vi "processing.vi"(0 "Refnum in":T2, 5 "manual crop":bool, 7 "Erode process":bool, 9 "invert":bool) -> (3 "height less than 1cm(80pixels)":bool, 4 "after complete processing":T2, 10 "array of mean":sgl[](array[numeric]), 14 "image features":T3, 15 "Array of SD":sgl[](array[numeric]))   [LabVIEW 2011]
uses:
  <vilib>/vision/Image Controls.llb/IMAQ Image.ctl
  <vilib>/vision/NI_Vision_Development_Module.lvlib
  <vilib>/Analysis/NI_AALBase.lvlib
panel:
  in  "Tab Control":T1(tab)
  out "after invert(optional), crop (optional)":T2(plugin-control)
  out "after theshold":T2(plugin-control)
  out "after scan and make text white":T2(plugin-control)
  out "after particle filter":T2(plugin-control)
  out "after b/w to gray":T2(plugin-control)
  in  "Look For (Threshold 1)":u32(ring) items=["Bright Objects", "Dark Objects"]
  in  "Keep/Remove Particles (Particle Filter 1)":bool=TRUE
  in  "Connectivity 4/8 (8) (Particle Filter 1)":bool=TRUE
  out "subarray":sgl[](array[numeric])
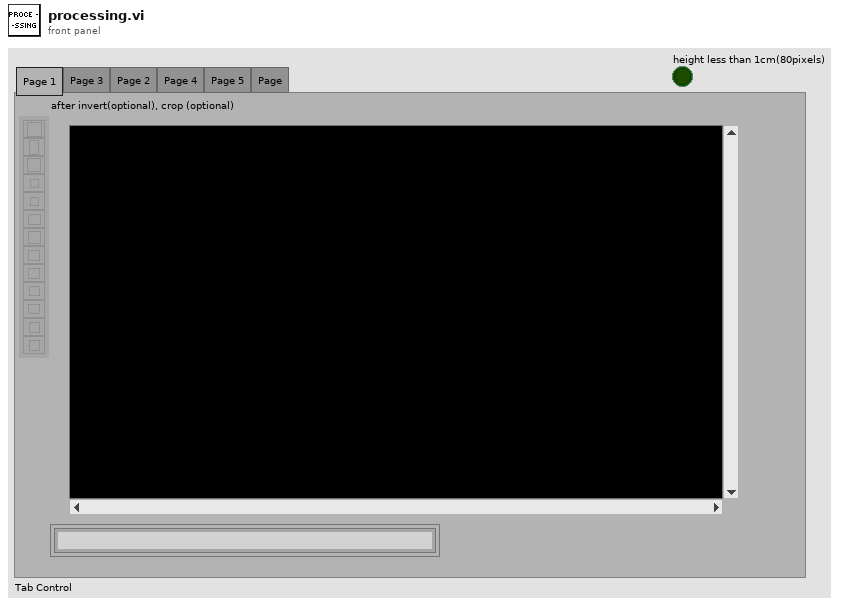
[diagram p1: front panel]
types:
  T1 = enum32{"Page 1", "Page 3", "Page 2", "Page 4", "Page 5", "Page"}
  T2 = typedef "IMAQ Image.ctl" = refnum<image>
  T3 = cluster{"text was :":bool, "top":i32, "bottom":i32}
  T4 = cluster{"Measurement Parameter":i32, "Range Lower Value":dbl, "Range Upper Value":dbl, "Range":bool, "Measurement Type":bool}[]
  T5 = enum32{"AutoM", "Close", "Dilate", "Erode", "Gradient", "Gradient in", "Gradient out", "HitMiss", "Open", "PClose", "POpen", "Thick", "Thin"}
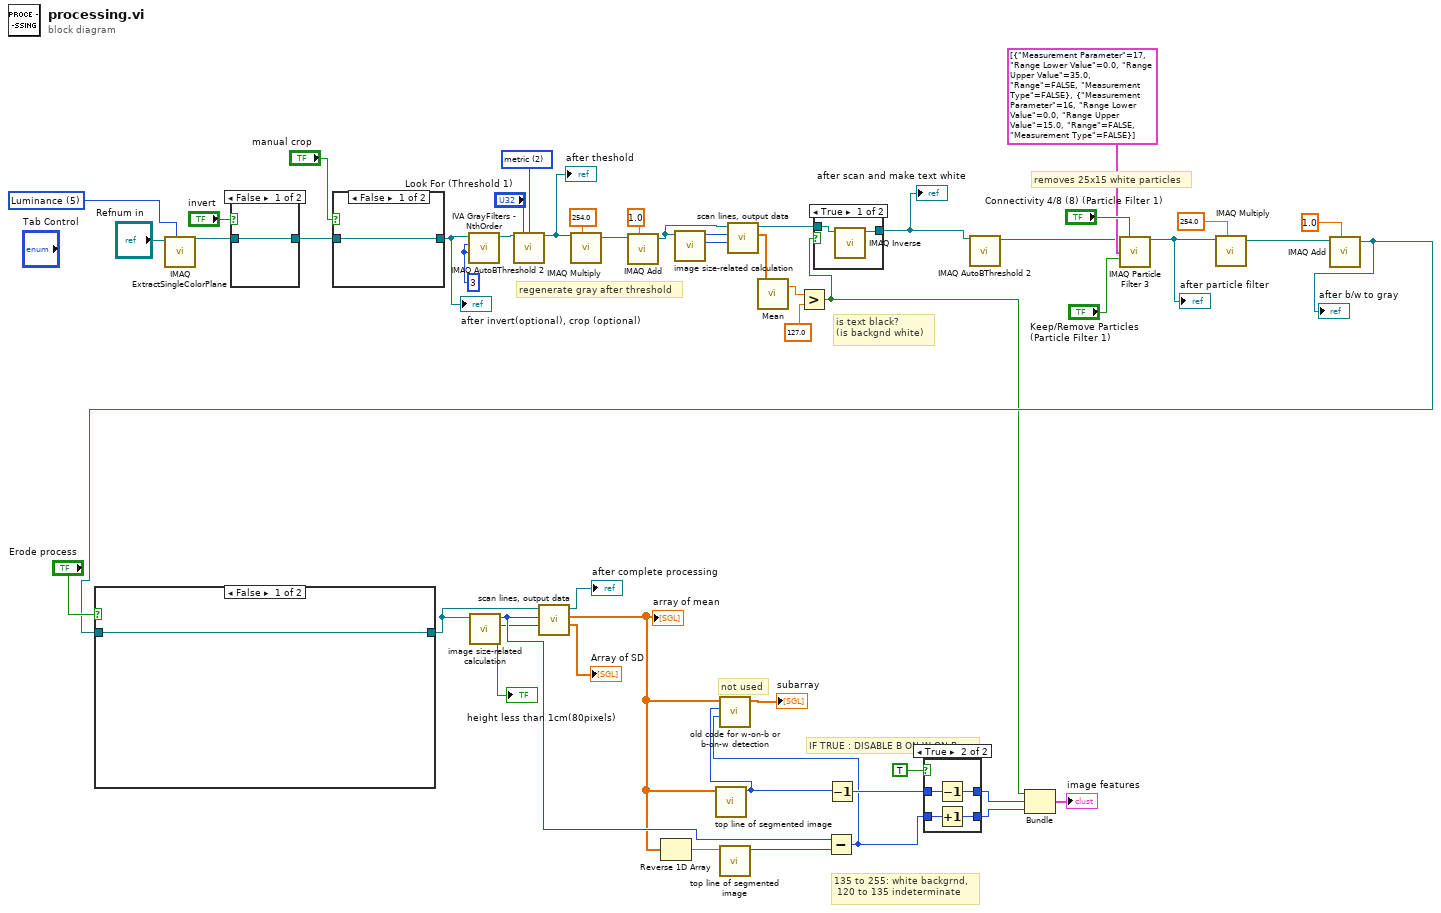
[diagram p0: block diagram]
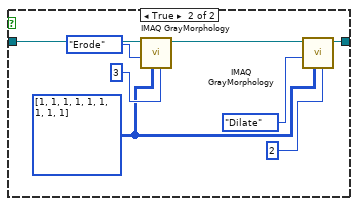
[diagram p4: hidden frame]
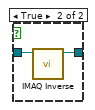
[diagram p5: hidden frame]
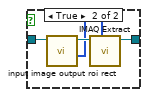
[diagram p6: hidden frame]
diagram:
  w37 = 3 ("Filter size X")
  w44 = 2 items=["clustering", "entropy", "metric", "moments", "inter-class variance"] ("Method (Threshold 1)")
  w47 = 5 items=["Red", "Green", "Blue", "Hue", "Saturation", "Luminance", "Value", "Intensity"] ("Color Plane (Color Plane Extraction 1)")
  # "not used"
  # "is text black?\n(is backgnd white)"
  # "regenerate gray after threshold"
  # "removes 25x15 white particles"
  # "IF TRUE : DISABLE B ON W ON B"
  # "135 to 255: white backgrnd,\n 120 to 135 indeterminate"
  n1 = call "IMAQ ExtractSingleColorPlane"("Color Plane"=w47, "Image Src"="Refnum in") -> ("Image Dst Out"=w49:T2)  [unwired: 2 in, 7 out]
  n2 = case shown="False" "invert" {
    tunnel: w49 -> [w52 w54]
    tunnel: [w52 w53] -> w46
    frame False {
    }
    frame True {
      n3 = call "IMAQ Inverse"("Image Src"=w54) -> ("Image Dst Out"=w53:T2)  [unwired: 9 in, 1 out]
    }
  }
  n4 = case shown="False" "manual crop" {
    tunnel: [w55 w58] -> w10
    tunnel: w46 -> [w55 w57]
    frame False {
    }
    frame True {
      n5 = call "input image output roi rect.vi"("Refnum in"=w57) -> ("selected rectangle"=w56:i32[], "Refnum out"=w59:T2)  [unwired: 9 in]
      n6 = call "IMAQ Extract"("Optional Rectangle"=w56, "Image Src"=w59) -> ("Image Dst Out"=w58:T2)  [unwired: 8 in, 1 out]
    }
  }
  "after invert(optional), crop (optional)" <- w10
  n7 = call <vilib>:"IVA GrayFilters - NthOrder.vi"("Filter size Y"=w37, "Filter size X"=w37, "Image In"=w10) -> ("Image Out"=w36:T2)  [unwired: 1 in, 7 out]
  n8 = call "IMAQ AutoBThreshold 2"("Image Src"=w36, "Look For (Bright Objects)"="Look For (Threshold 1)", "Method (clustering)"=w44) -> ("Image Dst Out"=w6:T2)  [unwired: 5 in, 7 out]
  "after theshold" <- w6
  n9 = call "IMAQ Multiply"("Image Src A"=w6, "Constant"=sgl 254.0) -> ("Image Dst Out"=w7:T2)  [unwired: 5 in, 1 out]
  n10 = call "IMAQ Add"("Image Src A"=w7, "Constant"=sgl 1.0) -> ("Image Dst Out"=w5:T2)  [unwired: 5 in, 1 out]
  n11 = call "image size-related calculation.vi"("Refnum in"=w5) -> ("width"=w18:i32, "no. of scanning lines"=w19:i32)  [unwired: 8 in, 1 out]
  n12 = call "scan lines, output data.vi"("width"=w18, "no. of scanning lines"=w19, "Refnum in"=w5) -> ("mean Array"=w15:sgl[], "Refnum out"=w12:T2)  [unwired: 6 in, 1 out]
  n13 = call <vilib>:"Mean.vi"("X"=w15) -> ("mean"=w16:dbl)  [unwired: 1 out]
  n14 = Greater?(x=w16, y=127.0) -> (0:w4:bool)
  n15 = case shown="True" w4 {
    tunnel: w12 -> [w61 w62]
    tunnel: [w60 w62] -> w3
    frame True {
      n16 = call "IMAQ Inverse"("Image Src"=w61) -> ("Image Dst Out"=w60:T2)  [unwired: 9 in, 1 out]
    }
    frame False {
    }
  }
  "after scan and make text white" <- w3
  n17 = call "IMAQ AutoBThreshold 2"("Image Src"=w3) -> ("Image Dst Out"=w2:T2)  [unwired: 7 in, 7 out]
  n18 = call "IMAQ Particle Filter 3"("Image Src"=w2, "Connectivity 4/8 (8)"="Connectivity 4/8 (8) (Particle Filter 1)", "Selection Values"=T4 [{"Measurement Parameter"=17, "Range Lower Value"=0.0, "Range Upper Value"=35.0, "Range"=FALSE, "Measurement Type"=FALSE}, {"Measurement Parameter"=16, "Range Lower Value"=0.0, "Range Upper Value"=15.0, "Range"=FALSE, "Measurement Type"=FALSE}] ("Selection Values (Particle Filter 1)"), "Keep/Remove Particles (F)"="Keep/Remove Particles (Particle Filter 1)") -> ("Image Dst Out"=w27:T2)  [unwired: 5 in, 6 out]
  "after particle filter" <- w27
  n19 = call "IMAQ Multiply"("Image Src A"=w27, "Constant"=sgl 254.0) -> ("Image Dst Out"=w41:T2)  [unwired: 5 in, 1 out]
  n20 = call "IMAQ Add"("Image Src A"=w41, "Constant"=sgl 1.0) -> ("Image Dst Out"=w26:T2)  [unwired: 5 in, 1 out]
  "after b/w to gray" <- w26
  n21 = case shown="False" "Erode process" {
    tunnel: [w63 w65] -> w39
    tunnel: w26 -> [w63 w64]
    frame False {
    }
    frame True {
      w66 = i32[][] [[1, 1, 1], [1, 1, 1], [1, 1, 1]] ("Structuring Element (Gray Morphology 1)")
      n22 = call "IMAQ GrayMorphology"("Number of iterations (1)"=3, "Structuring Element"=w66, "Operation"=T5."Erode" ("Operation (Gray Morphology 1)"), "Image Src"=w64) -> ("Image Dst Out"=w69:T2)  [unwired: 3 in, 4 out]
      n23 = call "IMAQ GrayMorphology"("Number of iterations (1)"=2, "Structuring Element"=w66, "Operation"=T5."Dilate", "Image Src"=w69) -> ("Image Dst Out"=w65:T2)  [unwired: 3 in, 4 out]
    }
  }
  n24 = call "image size-related calculation.vi"("Refnum in"=w39) -> ("height less than 1cm(80pixels)"=→"height less than 1cm(80pixels)":bool, "width"=w24:i32, "no. of scanning lines"=w25:i32)  [unwired: 8 in]
  n25 = call "scan lines, output data.vi"("width"=w24, "no. of scanning lines"=w25, "Refnum in"=w39) -> ("std dev arrays"=→"Array of SD":sgl[], "mean Array"=w20:sgl[], "Refnum out"=→"after complete processing":T2)  [unwired: 6 in]
  "array of mean" <- w20
  n26 = Reverse 1D Array(array=w20) -> (reversed array=w34:sgl[])
  n27 = call "top line of segmented image.vi"("Array"=w20) -> ("Numeric"=w22:i32)  [unwired: 10 in]
  n28 = call "top line of segmented image.vi"("Array"=w34) -> ("Numeric"=w33:i32)  [unwired: 10 in]
  n29 = Subtract(x=w25, y=w33) -> (x-y=w29:i32)
  n30 = call "old code for w-on-b or b-on-w detection.vi"("Numeric 2"=w29, "Numeric"=w22, "Array"=w20) -> ("subarray"=→"subarray":sgl[])  [unwired: 8 in]
  n31 = Decrement(x=w22) -> (x-1=w30:i32)
  n32 = case shown="True" TRUE {
    tunnel: [w73 w77] -> w32
    tunnel: w30 -> [w73 w76]
    tunnel: w29 -> [w72 w75]
    tunnel: [w72 w74] -> w28
    frame False {
    }
    frame True {
      n33 = Decrement(x=w76) -> (x-1=w77:i32)
      n34 = Increment(x=w75) -> (x+1=w74:i32)
    }
  }
  n35 = Bundle(w4, w32, w28) -> (→"image features":cluster{bool, i32, i32})  [unwired: 1 in]
